vi "SAPI Open Voice Object SubVI.vi"(8 "error in (no error)":errorcluster) -> (0 "error out":errorcluster, 1 "AudioOutputs":string[](array[string]), 2 "Voice Names":string[](array[string]), 3 "speech object references":T1)   [LabVIEW 2021, in "SAPI.TTS.lvlib"]
doc: "Opens a reference to the SAPI SpeechLib.ISpeechVoice object; returns lists of the available TTS voices and the available audio output devices. Returns a cluster of speech object references needed for each of the other SAPI TTS SubVIs."
uses:
  Users/sacha/Desktop/labview/TTS new 2012/SAPI TTS Library/SAPI.TTS.lvlib
  Users/sacha/Desktop/labview/TTS new 2012/SAPI TTS Library/Controls/Speech object references.ctl
panel:
  # "Opens a reference to the SAPI SpeechLib.ISpeechVoice object;\nreturns lists of the available TTS voices and the available audio\noutput devices. Returns a cluster of speech object references\nneeded for each of the other SAPI TTS SubVIs."
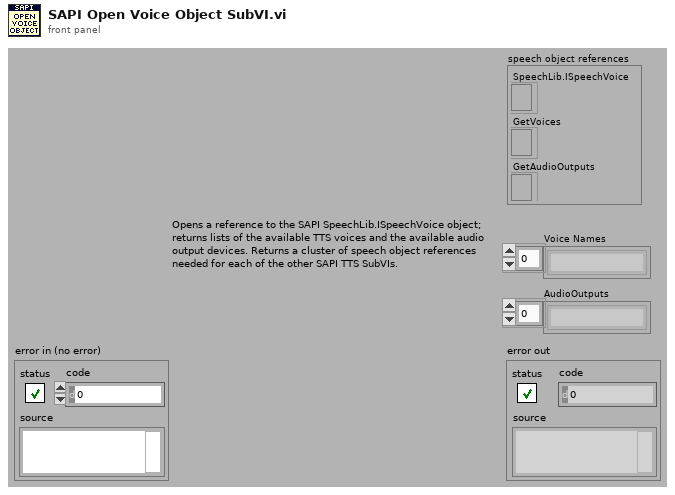
[diagram p1: front panel]
types:
  T1 = typedef "SAPI.TTS.lvlib/Speech object references.ctl" = cluster{"SpeechLib.ISpeechVoice":refnum<k7>, "GetVoices":refnum<k7>, "GetAudioOutputs":refnum<k7>}
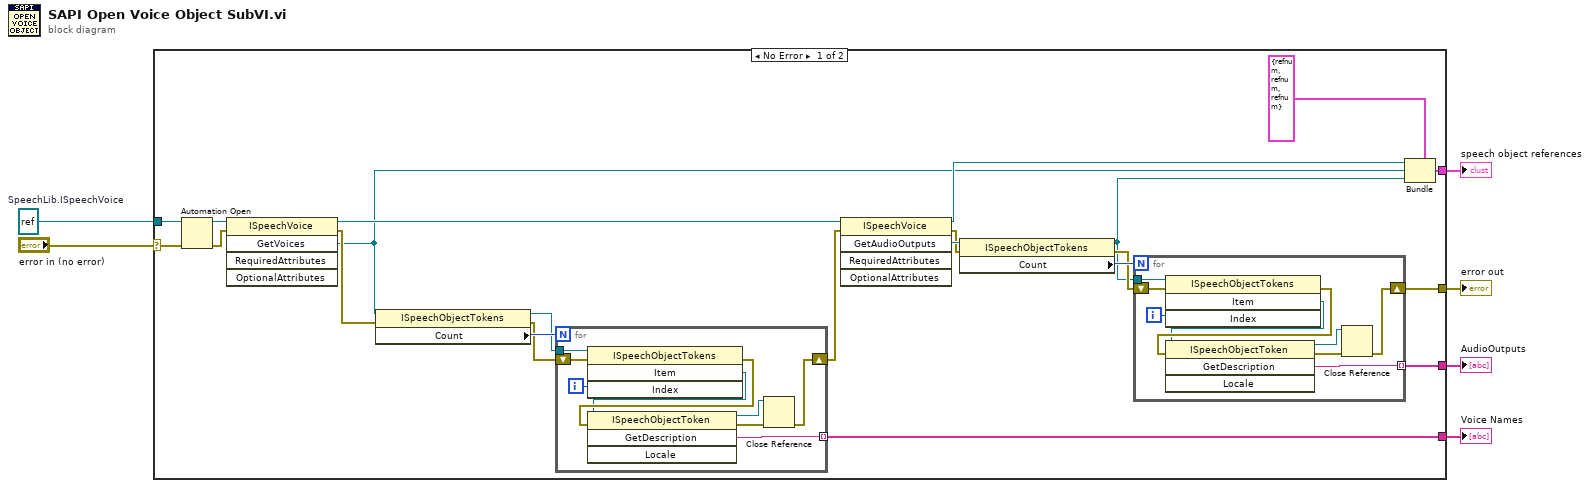
[diagram p0: block diagram]
diagram:
  w6 = refnum<k7> refnum  # SpeechLib.ISpeechVoice
  n1 = case shown="No Error" "error in (no error)" {
    selector: "error in (no error)" -> [w7 w47]
    tunnel: w6 -> [w28 _]
    tunnel: [w22 _] -> w5
    tunnel: [w14 w47] -> w4
    tunnel: [w13 _] -> w3
    tunnel: [w9 _] -> w2
    frame No Error {
      n2 = Automation Open(error in (no error)=w7, Automation Refnum=w28) -> (Automation Refnum=w25:refnum<k7>, error out=w21:errorcluster)  [unwired: 2 in]
      n3 = invoke class="ISpeechVoice" method="GetVoices"(reference=w25, error in=w21) -> (reference out=w20:refnum<k7>, error out=w26:errorcluster, "GetVoices"=w11:refnum<k7>)  [unwired: 3 in, 2 out]
      n4 = property class="ISpeechObjectTokens"(reference=w11, error in=w26) -> (reference out=w24:refnum<k7>, error out=w23:errorcluster, "Count"=w27:i32)
      n5 = for {
        N: w27 -> [_]
        tunnel: w24 -> [w44]
        tunnel: [w43] -> w22 mode=indexing
        shift-right: [w40] -> w17
        shift-left: w23 -> [w38]
        i -> [w46]
        n6 = invoke class="ISpeechObjectTokens" method="Item"(reference=w44, error in=w38, "Index"=w46) -> (error out=w42:errorcluster, "Item"=w39:refnum<k7>)  [unwired: 1 in, 2 out]
        n7 = invoke class="ISpeechObjectToken" method="GetDescription"(reference=w39, error in=w42) -> (reference out=w45:refnum<k7>, error out=w41:errorcluster, "GetDescription"=w43:string)  [unwired: 2 in, 1 out]
        n8 = Close Reference(reference=w45, error in (no error)=w41) -> (error out=w40:errorcluster)
      }
      n9 = invoke class="ISpeechVoice" method="GetAudioOutputs"(reference=w20, error in=w17) -> (reference out=w12:refnum<k7>, error out=w18:errorcluster, "GetAudioOutputs"=w19:refnum<k7>)  [unwired: 3 in, 2 out]
      n10 = property class="ISpeechObjectTokens"(reference=w19, error in=w18) -> (reference out=w10:refnum<k7>, error out=w15:errorcluster, "Count"=w16:i32)
      n11 = for {
        N: w16 -> [_]
        tunnel: w10 -> [w35]
        tunnel: [w34] -> w13 mode=indexing
        shift-right: [w31] -> w14
        shift-left: w15 -> [w29]
        i -> [w37]
        n12 = invoke class="ISpeechObjectTokens" method="Item"(reference=w35, error in=w29, "Index"=w37) -> (error out=w33:errorcluster, "Item"=w30:refnum<k7>)  [unwired: 1 in, 2 out]
        n13 = invoke class="ISpeechObjectToken" method="GetDescription"(reference=w30, error in=w33) -> (reference out=w36:refnum<k7>, error out=w32:errorcluster, "GetDescription"=w34:string)  [unwired: 2 in, 1 out]
        n14 = Close Reference(reference=w36, error in (no error)=w32) -> (error out=w31:errorcluster)
      }
      n15 = Bundle(cluster=T1 {"SpeechLib.ISpeechVoice"=refnum, "GetVoices"=refnum, "GetAudioOutputs"=refnum} ("speech object references"), "SpeechLib.ISpeechVoice"=w12, "GetVoices"=w11, "GetAudioOutputs"=w10) -> (w9:T1)
    }
    frame Error {
    }
  }
  "Voice Names" <- w5
  "error out" <- w4
  "AudioOutputs" <- w3
  "speech object references" <- w2
